vi "Find Best Cost Core.vi"(8 "error in (no error)":errorcluster, 10 "LRU Cache in":refnum<class "LRU Cache.lvclass">, 11 "State in":refnum<class "State.lvclass">) -> (0 "error out":errorcluster, 2 "LRU Cache out":refnum<class "LRU Cache.lvclass">, 3 "State out":refnum<class "State.lvclass">)   [LabVIEW 2019, in "23.lvlib" / "State.lvclass"]
uses:
  State.lvclass
  C:/Users/craig.walker/Documents/GitHub/lv2019-LRU-Cache/LRU Node/LRU Node.lvclass
  lv2019-LRU-Cache/LRU Cache/LRU Cache.lvclass
  lv2019-LRU-Cache/LRU Node/LRU Node.lvclass/LRU Node.ctl
  State Key/State Key.lvclass/State Key.ctl
  lv2019-LRU-Cache/LRU Cache/LRU Cache.lvclass/LRU Cache.ctl
  lv2019-Doubly-Linked-List/Doubly Linked List Node/Doubly Linked List Node.lvclass/Doubly Linked List Node.ctl
  lv2019-Doubly-Linked-List/Doubly Linked List/Doubly Linked List.lvclass/Doubly Linked List.ctl
  lv2019-LRU-Cache/LRU DLL/LRU DLL.lvclass/LRU DLL.ctl
  State Value/State Value.lvclass/State Value.ctl
  lv2019-LRU-Cache/LRU Node/Read Key.vi
  lv2019-LRU-Cache/LRU Cache/Check Hash Table.vi
  lv2019-LRU-Cache/LRU Cache/Move to Root.vi
  lv2019-LRU-Cache/LRU Cache/Add to Hash Table.vi
  lv2019-LRU-Cache/LRU Cache/Add to LRU DLL.vi
  lv2019-LRU-Cache/LRU Node/Create LRU DLL Node DVR.vi
  lv2019-LRU-Cache/LRU Cache/Remove from LRU DLL.vi
  lv2019-LRU-Cache/LRU Node/Destroy LRU Node DVR.vi
  lv2019-LRU-Cache/LRU Cache/Remove from Hash Table.vi
  lv2019-LRU-Cache/LRU Cache/Add to Decached Node Store.vi
  lv2019-LRU-Cache/LRU Node/Retrieve Node Value.vi
  lv2019-LRU-Cache/LRU Cache/Check Capacity.vi
  lv2019-LRU-Cache/LRU Cache/Check Detached Node Store.vi
  lv2019-LRU-Cache/LRU Node/Write Value.vi
  lv2019-LRU-Cache/LRU Node/Read Value.vi
  Read Rooms.vi
  lv2019-Doubly-Linked-List/Doubly Linked List/Move Node.vi
  lv2019-Doubly-Linked-List/Doubly Linked List/Add Node.vi
  lv2019-LRU-Cache/LRU DLL/Read Max Size.vi
  lv2019-LRU-Cache/LRU DLL/Read Size.vi
  lv2019-LRU-Cache/LRU DLL/Write Size.vi
  lv2019-Doubly-Linked-List/Doubly Linked List/Remove Tail.vi
  State Key/Read Rooms.vi
  lv2019-Doubly-Linked-List/Doubly Linked List/Remove Node.vi
  lv2019-Doubly-Linked-List/Doubly Linked List/Read Tail.vi
  lv2019-Doubly-Linked-List/Doubly Linked List/Write Tail.vi
  lv2019-Doubly-Linked-List/Doubly Linked List Node/Write Next.vi
  lv2019-Doubly-Linked-List/Doubly Linked List Node/Write Previous.vi
  lv2019-Doubly-Linked-List/Doubly Linked List/Write Root.vi
  lv2019-Doubly-Linked-List/Doubly Linked List/Read Root.vi
  lv2019-Doubly-Linked-List/Doubly Linked List Node/Read Next.vi
  lv2019-Doubly-Linked-List/Doubly Linked List/Search by Index.vi
  lv2019-Doubly-Linked-List/Doubly Linked List Node/Read Previous.vi
  lv2019-Doubly-Linked-List/Doubly Linked List/Root to Iterator.vi
  lv2019-LRU-Cache/LRU DLL/LRU DLL.lvclass
  C:/Users/craig.walker/Documents/GitHub/lv2019-Doubly-Linked-List/Doubly Linked List/Doubly Linked List.lvclass
  lv2019-LRU-Cache/LRU Node/LRU Node.lvclass
  C:/Users/craig.walker/Documents/GitHub/lv2019-Doubly-Linked-List/Doubly Linked List Node/Doubly Linked List Node.lvclass
  lv2019-Doubly-Linked-List/Doubly Linked List Node/Create DLL Node DVR.vi
  lv2019-Doubly-Linked-List/Doubly Linked List Node/Destroy DLL Node DVR.vi
  State Key/State Key.lvclass
  lv2019-Doubly-Linked-List/Doubly Linked List Node/Doubly Linked List Node.lvclass
  State Value/State Value.lvclass
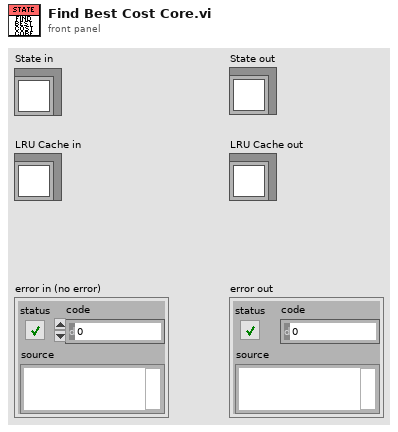
[diagram p1: front panel]
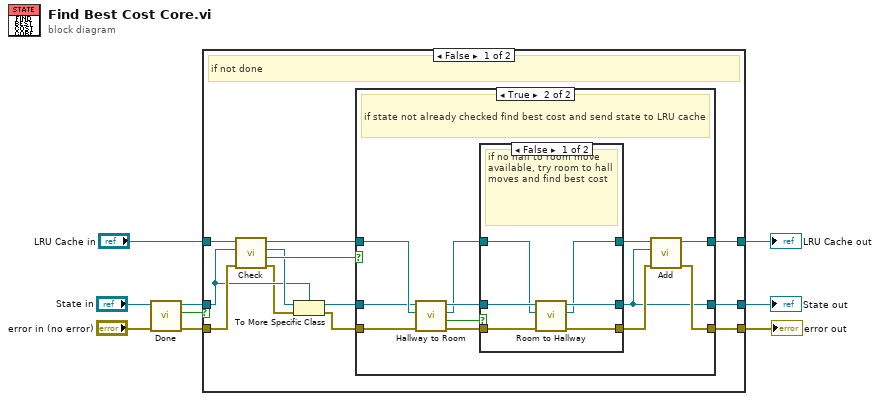
[diagram p0: block diagram]
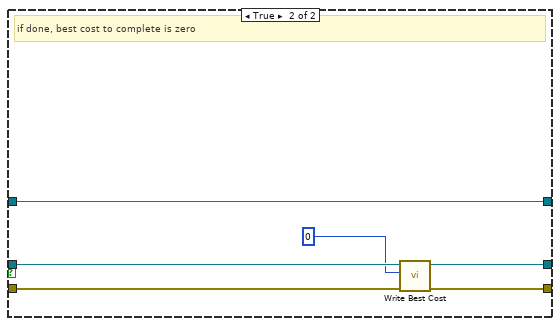
[diagram p4: hidden frame]
diagram:
  n1 = call "Done.vi"("error in (no error)"="error in (no error)", "State in"="State in") -> ("error out"=w4:errorcluster, "Done?"=w8:bool, "State out"=w7:refnum<class "State.lvclass">)  [unwired: 7 in]
  n2 = case shown="False" w8 {
    tunnel: w7 -> [w12 w50]
    tunnel: "LRU Cache in" -> [w21 w46]
    tunnel: w4 -> [w20 w48]
    tunnel: [w15 w51] -> w3
    tunnel: [w17 w46] -> w2
    tunnel: [w16 w47] -> w1
    frame False {
      # "if not done"
      n3 = call "Check.vi"("error in (no error)"=w20, "LRU Node in"=w12, "LRU Cache in"=w21) -> ("error out"=w11:errorcluster, "key not found?"=w19:bool, "LRU Node out"=w14:refnum<class "LRU Node.lvclass">, "LRU Cache out"=w18:refnum<class "LRU Cache.lvclass">)  [unwired: 5 in]
      n4 = To More Specific Class(target class=w12, reference=w14, error in=w11) -> (specific class reference=w13:refnum<class "State.lvclass">, error out=w10:errorcluster)
      n5 = case shown="True" w19 {
        tunnel: w13 -> [w24 w25]
        tunnel: w18 -> [w23 w32]
        tunnel: [w24 w26] -> w15
        tunnel: [w23 w29] -> w17
        tunnel: w10 -> [w22 w31]
        tunnel: [w22 w27] -> w16
        frame False {
          # "if state already checked pass state out"
        }
        frame True {
          # "if state not already checked find best cost and send state to LRU cache"
          n6 = call "Hallway to Room.vi"("error in (no error)"=w31, "LRU Cache in"=w32, "State in"=w25) -> ("error out"=w34:errorcluster, "Moved?"=w36:bool, "LRU Cache out"=w33:refnum<class "LRU Cache.lvclass">, "State out"=w35:refnum<class "State.lvclass">)  [unwired: 5 in]
          n7 = case shown="False" w36 {
            tunnel: w35 -> [w42 w45]
            tunnel: [w41 w45] -> w26
            tunnel: w34 -> [w37 w44]
            tunnel: [w40 w44] -> w28
            tunnel: w33 -> [w39 w43]
            tunnel: [w38 w43] -> w30
            frame False {
              # "if no hall to room move available, try room to hall moves and find best cost"
              n8 = call "Room to Hallway.vi"("error in (no error)"=w37, "LRU Cache in"=w39, "State in"=w42) -> ("error out"=w40:errorcluster, "LRU Cache out"=w38:refnum<class "LRU Cache.lvclass">, "State out"=w41:refnum<class "State.lvclass">)  [unwired: 6 in]
            }
            frame True {
              # "if moved from hall to room return best cost"
            }
          }
          n9 = call "Add.vi"("error in (no error)"=w28, "LRU Node"=w26, "LRU Cache in"=w30) -> ("error out"=w27:errorcluster, "LRU Cache out"=w29:refnum<class "LRU Cache.lvclass">)  [unwired: 7 in]
        }
      }
    }
    frame True {
      # "if done, best cost to complete is zero"
      n10 = call "Write Best Cost.vi"("error in (no error)"=w48, "Best Cost"=u64 0, "State in"=w50) -> ("error out"=w47:errorcluster, "State out"=w51:refnum<class "State.lvclass">)  [unwired: 7 in]
    }
  }
  "LRU Cache out" <- w2
  "State out" <- w3
  "error out" <- w1
